vi "API - CountUp Global.vi"() -> (3 "Data":i32)   [LabVIEW 2020]
uses:
  <userlib>/_NEVSTOP/Communicable State Machine(CSM)/_Support/Priority Queue/Priority Queue.lvclass/Priority Queue.ctl
  d9efecda-e120-4456-b024-2f9617889d36.vi
  <userlib>/_NEVSTOP/Communicable State Machine(CSM)/_Support/CSMQ/_Obtain CSM Data Queue.vi
  <userlib>/_NEVSTOP/Communicable State Machine(CSM)/_Support/Priority Queue/Release Priority Queue.vi
  <userlib>/_NEVSTOP/Communicable State Machine(CSM)/_Support/Process/CSMP-Sync Call.vi
  <userlib>/_NEVSTOP/Communicable State Machine(CSM)/Utility/uuid.vi
  <userlib>/_NEVSTOP/Communicable State Machine(CSM)/Utility/Build Error Cluster.vi
  <userlib>/_NEVSTOP/Communicable State Machine(CSM)/Utility/Trim Both Whitespace.vi
  <userlib>/_NEVSTOP/Communicable State Machine(CSM)/_Support/Priority Queue/Obtain Priority Queue.vi
  <userlib>/_NEVSTOP/Communicable State Machine(CSM)/_Support/CSMQ/_CSMObj-Message Check.vi
  <userlib>/_NEVSTOP/Communicable State Machine(CSM)/_Support/CSMQ/_CSMObj-Enqueue Cross-Module Message.vi
  <userlib>/_NEVSTOP/Communicable State Machine(CSM)/_Support/CSMQ/_CSMOFGV Get.vi
  <userlib>/_NEVSTOP/Communicable State Machine(CSM)/_Support/Priority Queue/Enqueue Element.vi
  <userlib>/_NEVSTOP/Communicable State Machine(CSM)/_Support/Error/CSM No Target Error.vi
  <userlib>/_NEVSTOP/Communicable State Machine(CSM)/_Support/CSMQ/_CSMOFGV.vi
  <userlib>/_NEVSTOP/Communicable State Machine(CSM)/_Support/Error/CSM Not Allowed Message.vi
  <userlib>/_NEVSTOP/Communicable State Machine(CSM)/_Support/Error/CSM Target Error.vi
  <userlib>/_NEVSTOP/Communicable State Machine(CSM)/_Support/Error/CSM Unhandled State Error.vi
  <userlib>/_NEVSTOP/Communicable State Machine(CSM)/_Support/Error/CSM Target Timeout Error.vi
  <userlib>/_NEVSTOP/Communicable State Machine(CSM)/addons/API-String-Arugments-Support/_Support/Convert API String Arguments to Data(variant).vi
  <userlib>/_NEVSTOP/Communicable State Machine(CSM)/_Support/Priority Queue/Priority Queue.lvclass
  <userlib>/_NEVSTOP/Communicable State Machine(CSM)/Communicable State Machine.lvlib
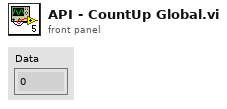
[diagram p1: front panel]
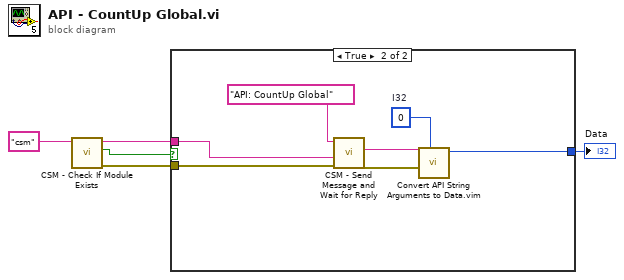
[diagram p0: block diagram]
diagram:
  n1 = call <userlib>:"CSM - Check If Module Exists.vi"("CSM Name"="csm") -> ("Error out"=w4:errorcluster, "Exist?"=w2:bool, "CSM Name(dup)"=w3:string)  [unwired: 8 in]
  n2 = case shown="True" w2 {
    tunnel: w4 -> [_ w12]
    tunnel: w3 -> [_ w11]
    tunnel: [_ w6] -> w1
    frame False {
    }
    frame True {
      w7 = 0  # I32
      n3 = call <userlib>:"CSM - Send Message and Wait for Reply.vi"("Error In (no error)"=w12, "Target Module"=w11, "State"="API: CountUp Global" ("CSM Name")) -> ("error out"=w9:errorcluster, "Response"=w8:string)  [unwired: 6 in, 1 out]
      n4 = call "Convert API String Arguments to Data.vim"("Type"=w7, "error in (no error)"=w9, "String"=w8) -> ("Data"=w6:i32)  [unwired: 5 in, 1 out]
    }
  }
  "Data" <- w1
